vi "SMU.SetOutput.vi"(8 "error in (no error)":errorcluster, 10 "Output (False)":bool, 11 "SMU in":refnum<class "SMU.lvclass">) -> (0 "error out":errorcluster, 3 "SMU out":refnum<class "SMU.lvclass">)   [LabVIEW 2017, in "SMU.lvclass"]
uses:
  SMU.lvclass
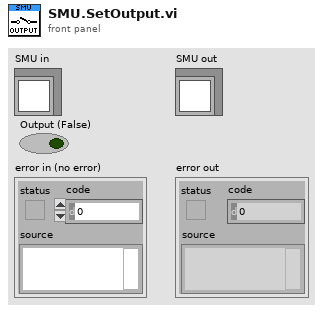
[diagram p1: front panel]
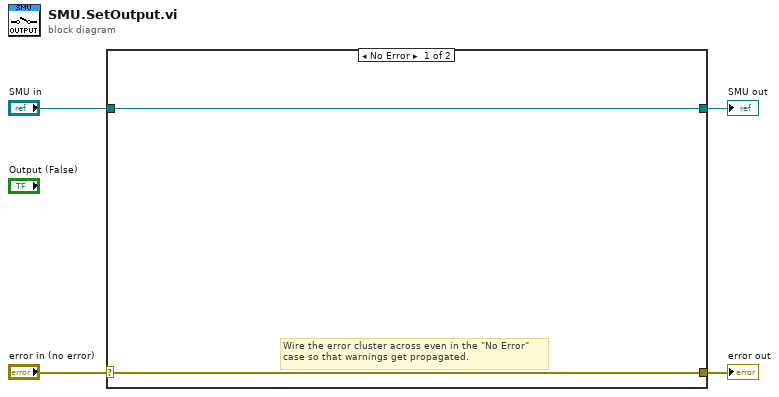
[diagram p0: block diagram]
diagram:
  n1 = case shown="No Error" "error in (no error)" {
    selector: "error in (no error)" -> [w5 w8]
    tunnel: [w5 w8] -> w3
    tunnel: [w6 w7] -> w1
    tunnel: "SMU in" -> [w6 w7]
    frame No Error {
      # "Wire the error cluster across even in the \"No Error\"\ncase so that warnings get propagated."
    }
    frame Error {
    }
  }
  "error out" <- w3
  "SMU out" <- w1
